vi "NXT-HID-Dual.vi"() -> ()   [LabVIEW 2009]
uses:
  <vilib>/NXT/Subs/LVHSConnector.ctl
  <vilib>/NXT/Block Support/NXT_InputPort.ctl
  mindsensors.com LVEE Toolkit/Dual/NXTHID-DM.vi
panel:
  out "Output of NXTHID":cluster{"Status (boolean)":bool}
  in  "Input of NXTHID":T1={"Transmit Mode"=1, "Text Data"="NXTHID is typing this...", "Key Modifier"=0, "Keydata"=58} {"Keydata" format="%x"; "Key Modifier" items=["None"=0, "Left Control"=1, "Left Shift"=2, "Left Alt"=4, "Left GUI"=8, "Right Control"=16, "Right Shift"=32, "Right Alt"=64, "Right GUI"=-128]; "Transmit Mode" items=["Direct Keyboard data", "Ascii Text data"]}
  in  "Input Port":T2 items=["Port 1", "Port 2", "Port 3", "Port 4"]
  out "NXT dup":T3={"error"={"status"=FALSE, "code"=0, "source"=""}, "address"="", "NXT #"=-1, "Show Error"=TRUE}
  in  "NXT":T3={"error"={"status"=FALSE, "code"=0, "source"=""}, "address"="", "NXT #"=-1, "Show Error"=TRUE}
  # "mindsensors.com\nCopyright (c) 2009 by mindsensors.com\nEmail: info (<at>) mindsensors (<dot>) com\n\nThis program is free software. You can redistribute it and/or modify\nit under the terms of the GNU General Public License as published by\nthe Free Software Foundation; version 3 of the License.\nRead the license at: http://www.gnu.org/licenses/gpl.txt"
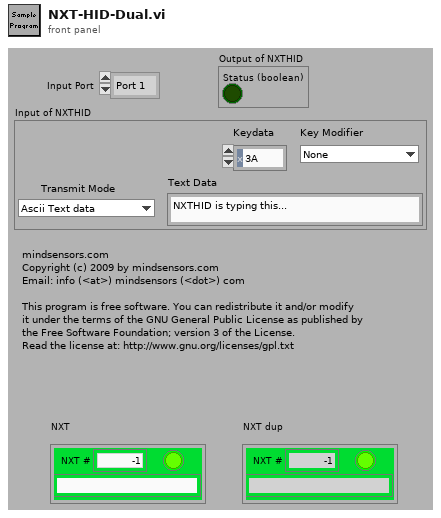
[diagram p1: front panel]
types:
  T1 = cluster{"Transmit Mode":u8, "Text Data":string, "Key Modifier":i8, "Keydata":u8}
  T2 = typedef "NXT_InputPort.ctl" = u8
  T3 = typedef "LVHSConnector.ctl" = cluster{"error":errorcluster, "address":string, "NXT #":i32, "Show Error":bool}
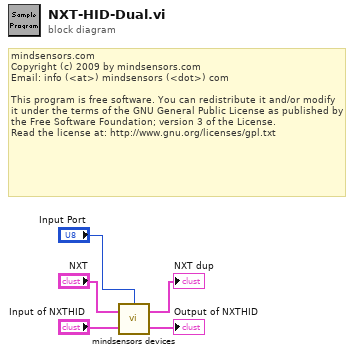
[diagram p0: block diagram]
diagram:
  # "mindsensors.com\nCopyright (c) 2009 by mindsensors.com\nEmail: info (<at>) mindsensors (<dot>) com\n\nThis program is free software. You can redistribute it and/or modify\nit under the terms of the GNU General Public License as published by\nthe Free Software Foundation; version 3 of the License.\nRead the license at: http://www.gnu.org/licenses/gpl.txt"
  n1 = call-poly "mindsensors devices.vi"("Input of NXTHID"="Input of NXTHID", "NXT"="NXT", "Input Port"="Input Port") -> ("Output of NXTHID"=→"Output of NXTHID":cluster{"Status (boolean)":bool}, "NXT dup"=→"NXT dup":T3)
